vi "【实际】1个数据采集模块1个被击打部位1次击打.vi"() -> ()   [LabVIEW 2010]
uses:
  <vilib>/Waveform/WDTFileIO.llb/Export Waveform To Spreadsheet File.vi
  DMP401-LabVIEW/DMP401-LabVIEW/DMP401.dll
panel:
  out "Y max":dbl caption="Y最大" format="%0.2f"
  out "AD值图表":dbl(graph)
  out "反应时间（秒）":u32
  in  "设备号":u8
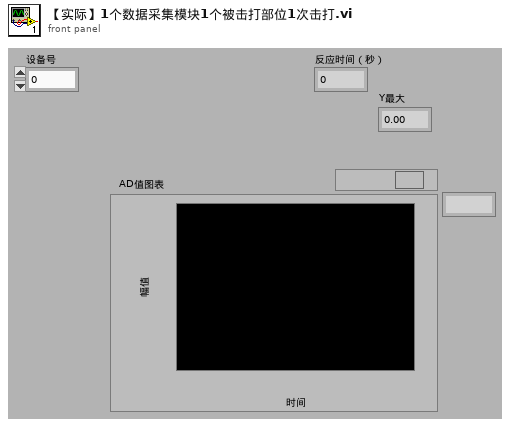
[diagram p1: front panel]
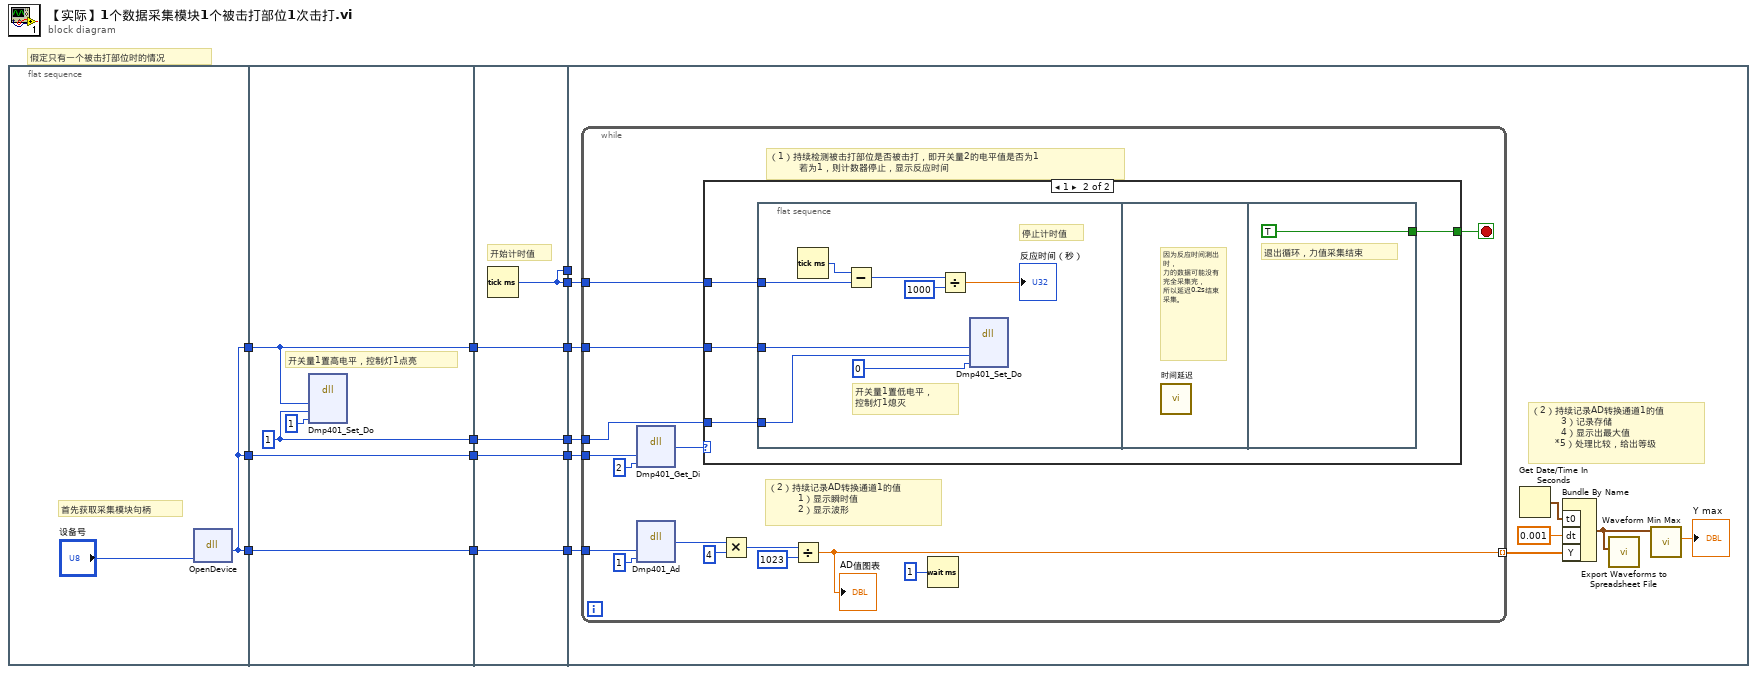
[diagram p0: block diagram]
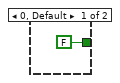
[diagram p2: hidden frame]
diagram:
  # "假定只有一个被击打部位时的情况"
  n1 = flat-sequence {
    tunnel: [w14] -> w13
    tunnel: [w14] -> w10
    tunnel: [w14] -> w6
    tunnel: w13 -> [w17]
    tunnel: [w19] -> w11
    tunnel: w10 -> [w19]
    tunnel: [w18] -> w7
    tunnel: w6 -> [w18]
    tunnel: [w17] -> w3
    tunnel: [w16] -> w2
    tunnel: [w25] -> w12
    tunnel: w11 -> [w25]
    tunnel: [w23] -> w9
    tunnel: [w24] -> w8
    tunnel: w7 -> [w24]
    tunnel: [w23] -> w5
    tunnel: [w22] -> w4
    tunnel: w3 -> [w22]
    tunnel: w2 -> [w21]
    tunnel: [w21] -> w1
    tunnel: w12 -> [w35]
    tunnel: w9 -> [w34]
    tunnel: w8 -> [w33]
    tunnel: w5 -> [_]
    tunnel: w4 -> [w27]
    tunnel: w1 -> [w26]
    frame #0 {
      # "首先获取采集模块句柄"
      n2 = dll-call lib="H:/Users/冯逸飞/Desktop/201107科研/DMP401-LabVIEW/DMP401-LabVIEW/DMP401.dll" fn="OpenDevice"("设备号"="设备号") -> ("模块句柄（返回值）"=w14:u64)  [unwired: 4 in, 2 out]
    }
    frame #1 {
      w16 = u8 1 ("开关量通道号")
      # "开关量1置高电平，控制灯1点亮"
      n3 = dll-call lib="H:/Users/冯逸飞/Desktop/201107科研/DMP401-LabVIEW/DMP401-LabVIEW/DMP401.dll" fn="Dmp401_Set_Do"("模块句柄"=w17, "开关量通道号"=w16, "开关量值"=u8 1) -> ()  [unwired: 7 in, 2 out]
    }
    frame #2 {
      # "开始计时值"
      n4 = Tick Count (ms)() -> (millisecond timer value=w23:u32)
    }
    frame #3 {
      # "（2）持续记录AD转换通道1的值\n          3）记录存储\n          4）显示出最大值\n        *5）处理比较，给出等级"
      n5 = while {
        tunnel: w35 -> [w50]
        tunnel: w34 -> [w47]
        tunnel: w33 -> [w45]
        tunnel: [w38] -> w29 mode=indexing
        tunnel: w27 -> [w37]
        tunnel: w26 -> [w36]
        stop <- w46 stop-if-true
        # "（2）持续记录AD转换通道1的值\n          1）显示瞬时值\n          2）显示波形"
        # "（1）持续检测被击打部位是否被击打，即开关量2的电平值是否为1\n          若为1，则计数器停止，显示反应时间"
        n6 = dll-call lib="H:/Users/冯逸飞/Desktop/201107科研/DMP401-LabVIEW/DMP401-LabVIEW/DMP401.dll" fn="Dmp401_Get_Di"("模块句柄"=w50, "开关量通道号"=u8 2) -> ("开关量2电平值"=w48:u8)  [unwired: 5 in, 2 out]
        n7 = dll-call lib="H:/Users/冯逸飞/Desktop/201107科研/DMP401-LabVIEW/DMP401-LabVIEW/DMP401.dll" fn="Dmp401_Ad"("模块句柄"=w45, "AD通道号"=u8 1) -> ("AD值"=w44:u16)  [unwired: 5 in, 2 out]
        n8 = case shown="1" w48 {
          tunnel: w47 -> [_ w55]
          tunnel: [FALSE w54] -> w46
          tunnel: w37 -> [_ w53]
          tunnel: w36 -> [_ w52]
          frame 0, Default {
          }
          frame 1 {
            n9 = flat-sequence {
              tunnel: w55 -> [w62]
              tunnel: w53 -> [w57]
              tunnel: w52 -> [w56]
              tunnel: [TRUE] -> w54
              frame #0 {
                # "开关量1置低电平，\n控制灯1熄灭"
                # "停止计时值"
                n10 = Tick Count (ms)() -> (millisecond timer value=w63:u32)
                n11 = Subtract(x=w63, y=w62) -> (x-y=w61:u32)
                n12 = Divide(x=w61, y=u32 1000) -> (x/y=→"反应时间（秒）":dbl)
                n13 = dll-call lib="H:/Users/冯逸飞/Desktop/201107科研/DMP401-LabVIEW/DMP401-LabVIEW/DMP401.dll" fn="Dmp401_Set_Do"("模块句柄"=w57, "开关量通道号"=w56, "开关量值"=u8 0) -> ()  [unwired: 7 in, 2 out]
              }
              frame #1 {
                # "因为反应时间测出时，\n力的数据可能没有完全采集完，\n所以延迟0.2s结束采集。"
                n14 = call "时间延迟"() -> ()  [unwired: 11 in, 1 out]
              }
              frame #2 {
                # "退出循环，力值采集结束"
              }
            }
          }
        }
        n15 = Multiply(x=w44, y=u16 4) -> (x*y=w42:u16)
        n16 = Divide(x=w42, y=u16 1023) -> (x/y=w38:dbl)
        "AD值图表" <- w38
        n17 = Wait (ms)(milliseconds to wait=u32 1 ("等待时间（毫秒）")) -> ()  [unwired: 1 out]
      }
      n18 = Get Date/Time In Seconds() -> (seconds since 1Jan1904=w32:timestamp)
      n19 = Bundle By Name("t0"=w32, "dt"=0.001, "Y"=w29) -> (w28:waveform(dbl))  [unwired: 1 in]
      n20 = call-poly <vilib>:"Export Waveforms to Spreadsheet File.vi"("waveform"=w28) -> ()  [unwired: 9 in, 2 out]
      n21 = call <vilib>:"Waveform Min Max.vi"("waveform in"=w28) -> ("Y max"=→"Y max":dbl)  [unwired: 5 in, 5 out]
    }
  }
